vi "Validate Connection (with Reconnect).vi"(8 "error in (no error)":errorcluster, 11 "LV-Data.PGSQL in":refnum<class "LV-Data.PGSQL.lvclass">) -> (0 "error out":errorcluster, 3 "LV-Data.PGSQL out":refnum<class "LV-Data.PGSQL.lvclass">)   [LabVIEW 2019, in "LV-Data.PGSQL.lvclass"]
uses:
  LV-Data.PGSQL.lvclass
  <vilib>/JDP Science/PostgreSQL Library/Connection/PQ Connection.lvclass
  LV-Data.PGSQL.lvclass/LV-Data.PGSQL.ctl
  <vilib>/JDP Science/PostgreSQL Library/Result/PQ Result.lvclass/PQ Result.ctl
  <vilib>/JDP Science/PostgreSQL Library/Connection/Execute Command (string result).vi
  <vilib>/JDP Science/PostgreSQL Library/Result/Get Column String.vi
  <vilib>/JDP Science/PostgreSQL Library/Result/subVIs/PQ DVR Error.vi
  <vilib>/JDP Science/PostgreSQL Library/Connection/Execute Command (Result).vi
  <vilib>/Utility/error.llb/Error Cluster From Error Code.vi
  <vilib>/JDP Science/PostgreSQL Library/Result/Clear.vi
panel:
  out "String":string
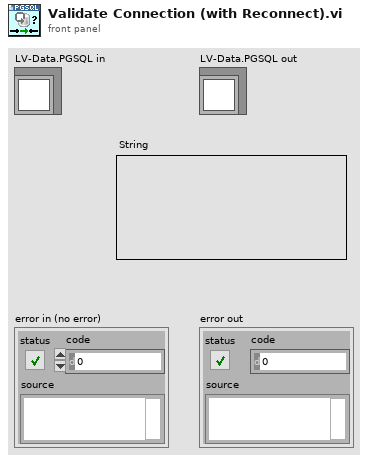
[diagram p1: front panel]
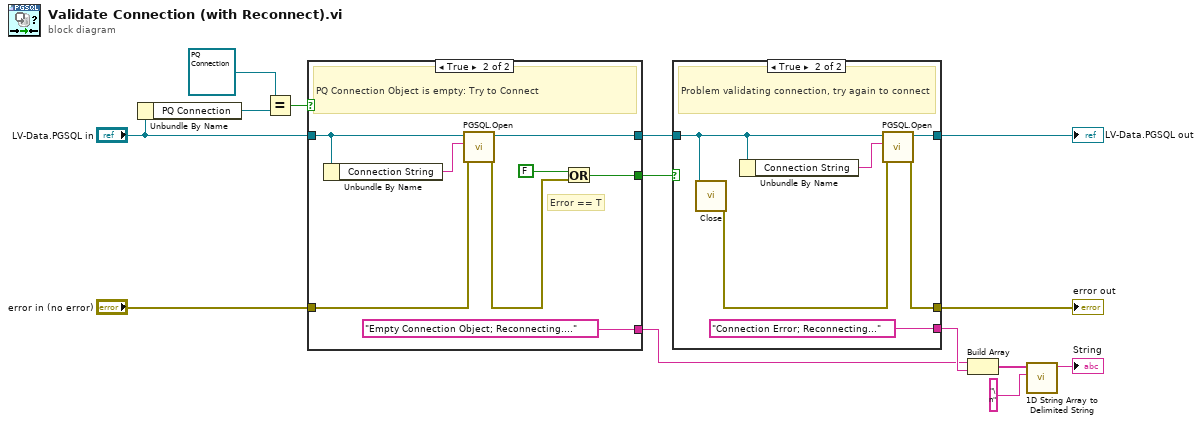
[diagram p0: block diagram]
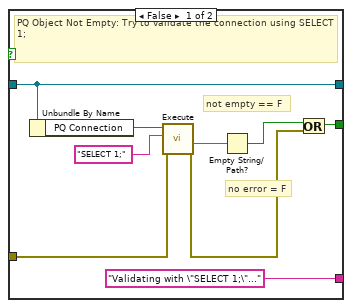
[diagram p2: hidden frame]
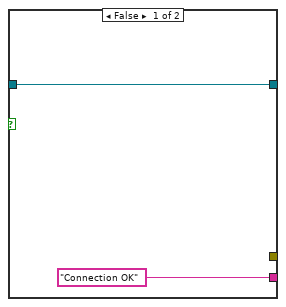
[diagram p3: hidden frame]
diagram:
  n1 = Unbundle By Name("LV-Data.PGSQL in") -> ("PQ Connection"=w7:refnum<class "PQ Connection.lvclass">)
  n2 = Equal?(x=refnum<class "PQ Connection.lvclass"> refnum ("PQ Connection"), y=w7) -> (x = y?=w8:bool)
  n3 = case shown="True" w8 {
    tunnel: "LV-Data.PGSQL in" -> [w21 w30]
    tunnel: [w21 w31] -> w13
    tunnel: "error in (no error)" -> [w20 w29]
    tunnel: [w18 w26] -> w14
    tunnel: ["Validating with \"SELECT 1;\"..." "Empty Connection Object; Reconnecting...."] -> w1
    frame False {
      # "not empty == F"
      # "no error = F"
      # "PQ Object Not Empty: Try to validate the connection using SELECT 1;"
      n4 = Unbundle By Name(w21) -> ("PQ Connection"=w23:refnum<class "PQ Connection.lvclass">)
      n5 = call-poly <vilib>:"Execute.vi"("error in (no error)"=w20, "SQL"="SELECT 1;", "PQ Connection in"=w23) -> ("error out"=w17:errorcluster, "Result"=w19:string)  [unwired: 6 in, 1 out]
      n6 = Empty String/Path?(string/path=w19) -> (empty?=w16:bool)
      n7 = Or(x=w16, y=w17) -> (x .or. y?=w18:bool)
    }
    frame True {
      # "Error == T"
      # "PQ Connection Object is empty: Try to Connect"
      n8 = Unbundle By Name(w30) -> ("Connection String"=w28:string)
      n9 = call "PGSQL.Open.vi"("error in (no error)"=w29, "Connection String"=w28, "Data.PG in"=w30) -> ("error out"=w25:errorcluster, "Data.PG out"=w31:refnum<class "LV-Data.PGSQL.lvclass">)  [unwired: 7 in]
      n10 = Or(x=FALSE, y=w25) -> (x .or. y?=w26:bool)
    }
  }
  n11 = case shown="True" w14 {
    tunnel: [w33 w38] -> w11
    tunnel: w13 -> [w33 w37]
    tunnel: [_ w35] -> w12
    tunnel: ["Connection OK" "Connection Error; Reconnecting..."] -> w2
    frame False {
    }
    frame True {
      # "Problem validating connection, try again to connect"
      n12 = call-dynamic "Close.vi"("Data.PG in"=w37) -> ("error out"=w36:errorcluster)  [unwired: 9 in, 1 out]
      n13 = Unbundle By Name(w37) -> ("Connection String"=w39:string)
      n14 = call "PGSQL.Open.vi"("error in (no error)"=w36, "Connection String"=w39, "Data.PG in"=w37) -> ("error out"=w35:errorcluster, "Data.PG out"=w38:refnum<class "LV-Data.PGSQL.lvclass">)  [unwired: 7 in]
    }
  }
  "error out" <- w12
  "LV-Data.PGSQL out" <- w11
  n15 = Build Array(w1, w2) -> (w5:string[])
  n16 = call <vilib>:"1D String Array to Delimited String.vi"("delimiter"="\n", "string array"=w5) -> ("delimited string"=→"String":string)  [unwired: 9 in]
